vi "Tacuri Victor_Autotronica_LabView.vi"() -> ()   [LabVIEW 2025]
uses:
  <vilib>/express/express arith-compare/Formula/XNode/ExpressFormulaBlockNode.xnode
panel:
  in  "stop":bool
  out "Fahrenheit":dbl
  out "Fahrenheit":dbl(knob) scale=0.0..10.0
  out "Kelvin":dbl
  out "Kelvin":dbl(knob) scale=0.0..10.0
  out "Celsius":dbl(knob) scale=0.0..10.0
  out "Celsisu":dbl
  out "Led frio":bool
  out "Led caliente":bool
  out "Kelvin":dbl(slide) scale=0.0..100.0
  out "Fahrenheit":dbl(slide) scale=0.0..100.0
  in  "Slide":dbl(slide) scale=0.0..100.0
  out "Celsius":dbl(slide) scale=0.0..100.0
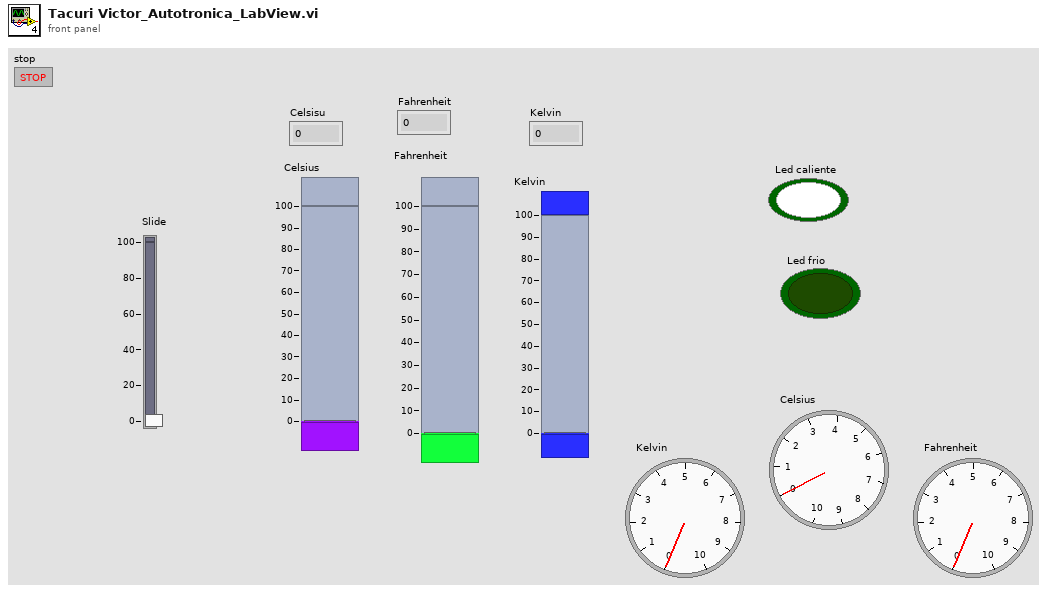
[diagram p1: front panel]
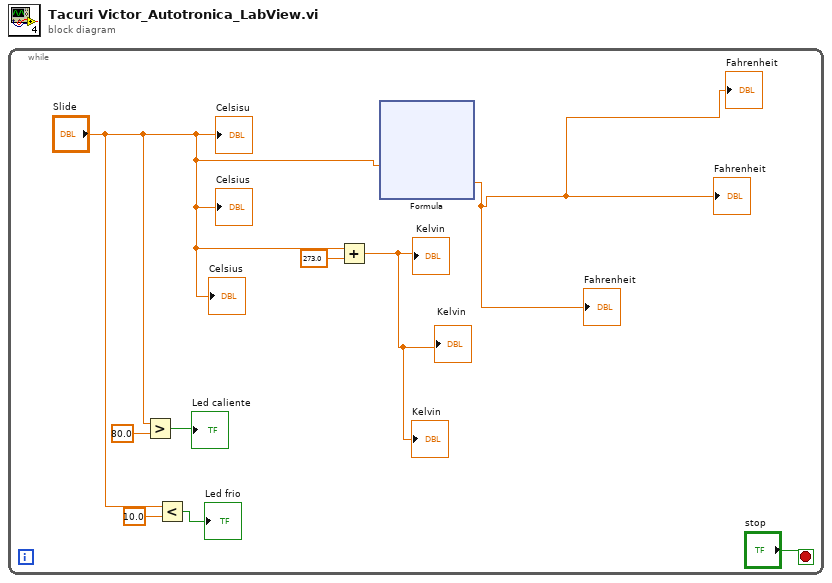
[diagram p0: block diagram]
diagram:
  n1 = while {
    stop <- "stop" stop-if-true
    n2 = Greater?(x="Slide", y=80.0) -> (0:→"Led caliente":bool)
    n3 = Less?(x="Slide", y=10.0) -> (x < y?=→"Led frio":bool)
    n4 = Add(x="Slide", y=273.0) -> (x+y=→"Kelvin" →"Kelvin" →"Kelvin":dbl)
    n5 = xnode "Formula"("X1"="Slide") -> ("Result"=→"Fahrenheit" →"Fahrenheit" →"Fahrenheit":dbl)  [unwired: 1 in, 1 out]
    "Celsius" <- "Slide"
    "Celsisu" <- "Slide"
    "Celsius" <- "Slide"
  }
